vi "Generate Error.vi"(6 "hierarchy skip (1)":i32=1, 7 "show call chain? (T)":bool=TRUE, 8 "error in (no error)":errorcluster, 10 "error message":string, 11 "error code":i32) -> (0 "error out":errorcluster)   [LabVIEW 2020, in "CTI.lvlib"]
uses:
  CTI.lvlib
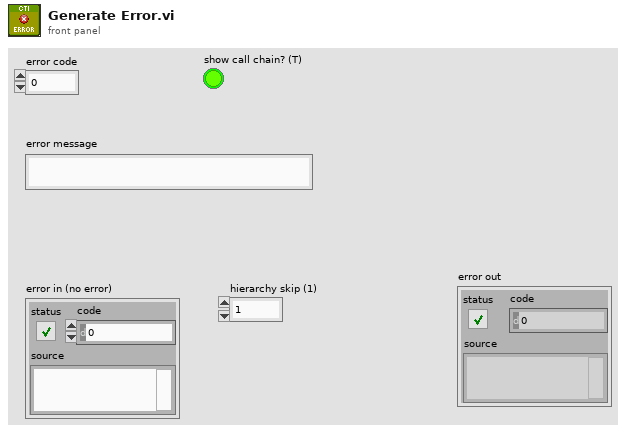
[diagram p1: front panel]
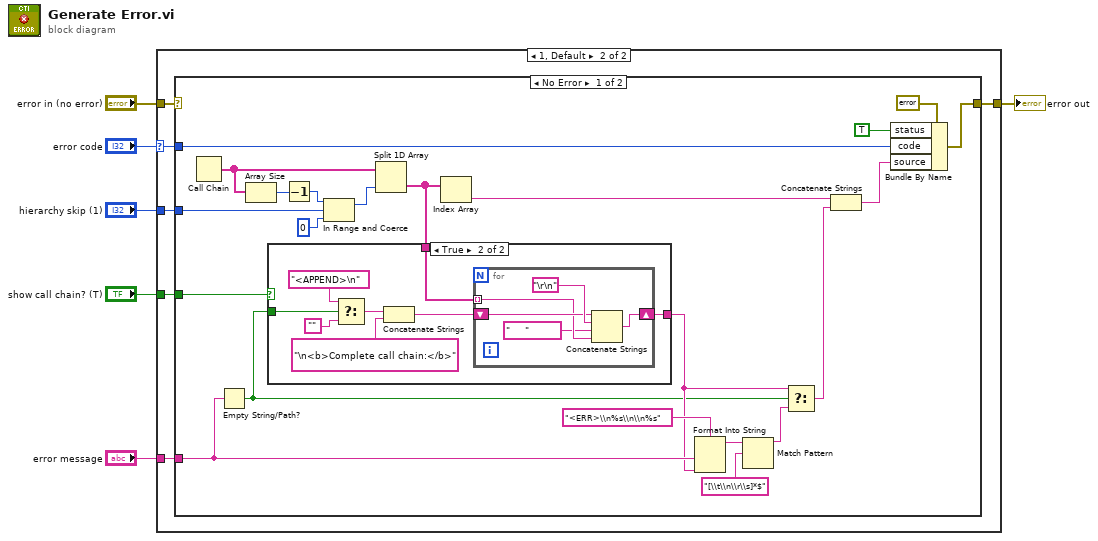
[diagram p0: block diagram]
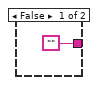
[diagram p3: hidden frame]
diagram:
  n1 = case shown="1, Default" "error code" {
    selector: "error code" -> [_ w11]
    tunnel: [w7 w13] -> w1
    tunnel: "error in (no error)" -> [w7 w12]
    tunnel: "error message" -> [_ w10]
    tunnel: "show call chain? (T)" -> [_ w9]
    tunnel: "hierarchy skip (1)" -> [_ w8]
    frame 0 {
      # "If the error code in equals zero, then propagate the error in cluster regardless of its value."
    }
    frame 1, Default {
      n2 = case shown="No Error" w12 {
        selector: w12 -> [_ w50]
        tunnel: [w35 w50] -> w13
        tunnel: w11 -> [w34 _]
        tunnel: w10 -> [w33 _]
        tunnel: w9 -> [w32 _]
        tunnel: w8 -> [w19 _]
        frame No Error {
          n3 = Call Chain() -> (call chain=w16:string[])
          n4 = Empty String/Path?(string/path=w33) -> (empty?=w26:bool)
          n5 = Array Size(array=w16) -> (size(s)=w20:i32)
          n6 = Decrement(x=w20) -> (x-1=w17:i32)
          n7 = In Range and Coerce(upper limit=w17, x=w19, lower limit=0) -> (coerced(x)=w15:i32)  [unwired: 1 out]
          n8 = Split 1D Array(array=w16, index=w15) -> (second subarray=w14:string[])  [unwired: 1 out]
          n9 = case shown="True" w32 {
            tunnel: ["" w44] -> w28
            tunnel: w26 -> [_ w41]
            tunnel: w14 -> [_ w37]
            frame False {
            }
            frame True {
              n10 = Select(t="<APPEND>\n", s=w41, f="") -> (s? t:f=w38:string)
              n11 = Concatenate Strings(w38, "\n<b>Complete call chain:</b>" ("call chain header")) -> (w42:string)
              n12 = for {
                tunnel: w37 -> [w46] mode=indexing
                shift-right: [w49] -> w44
                shift-left: w42 -> [w47]
                n13 = Concatenate Strings(w47, "\r\n", "     ", w46) -> (w49:string)
              }
            }
          }
          n14 = Index Array(array=w14) -> (element=w22:string)  [unwired: 1 in]
          n15 = Format Into String(format string="<ERR>\\n%s\\n\\n%s", w33, w28) -> (resulting string=w24:string)  [unwired: 2 in, 1 out]
          n16 = Match Pattern(string=w24, regular expression="[\\t\\n\\r\\s]*$") -> (before substring=w23:string)  [unwired: 1 in, 3 out]
          n17 = Select(t=w28, s=w26, f=w23) -> (s? t:f=w27:string)
          n18 = Concatenate Strings(w22, w27) -> (w30:string)
          n19 = Bundle By Name(cluster=errorcluster {"status"=FALSE, "code"=0, "source"=""} ("error out"), "status"=TRUE, "code"=w34, "source"=w30) -> (w35:errorcluster)
        }
        frame Error {
          # "An error in trumps any error code input."
        }
      }
    }
  }
  "error out" <- w1
